vi "Write Child Items.vi"(8 "error in":errorcluster, 10 "Child Items":cluster{"Type":T1, "Value":variant}[](array[cluster]), 11 "Item in":refnum<class "Item.lvclass">) -> (0 "error out":errorcluster, 3 "Item out":refnum<class "Item.lvclass">)   [LabVIEW 2024, in "Config File Parser.lvlib" / "Item.lvclass"]
uses:
  Item.lvclass
  Item Type.ctl
  Item.lvclass/Item.ctl
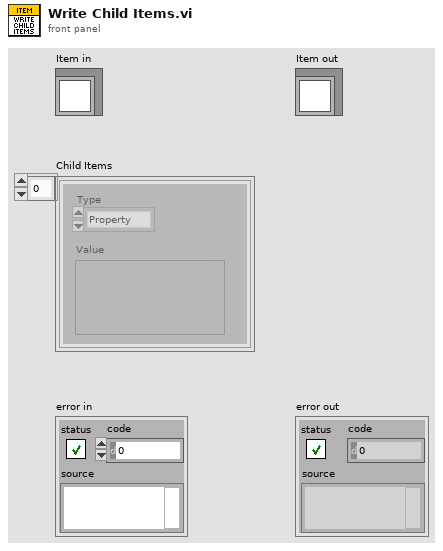
[diagram p1: front panel]
types:
  T1 = typedef "Config File Parser.lvlib/Item.lvclass/Item Type.ctl" = enum16{"Property", "Channel", "Section"}
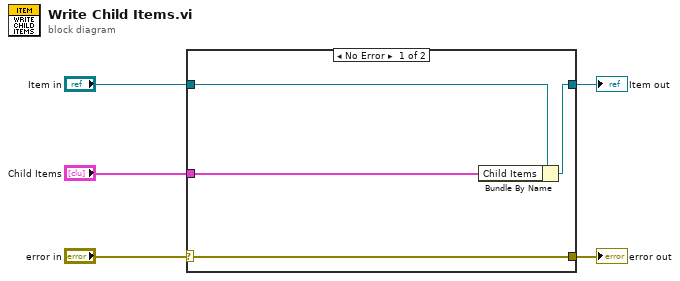
[diagram p0: block diagram]
diagram:
  n1 = case shown="No Error" "error in" {
    selector: "error in" -> [w9 w11]
    tunnel: [w9 w11] -> w4
    tunnel: [w7 w10] -> w2
    tunnel: "Item in" -> [w8 w10]
    tunnel: "Child Items" -> [w6 _]
    frame No Error {
      n2 = Bundle By Name(cluster=w8, "Child Items"=w6) -> (w7:refnum<class "Item.lvclass">)
    }
    frame Error {
    }
  }
  "error out" <- w4
  "Item out" <- w2
